vi "pl1000SetInterval.vi"(0 "pl1000 handle":i16, 5 "usForBlock":u32, 7 "idealNoOfSamples":u32, 9 "channels":i16[](array[numeric]), 11 "error in (no error)":errorcluster) -> (4 "pl1000 handle out":i16, 6 "usForBlock OP":u32, 8 "idealNoOfSamples OP":u32, 15 "error out":errorcluster)   [LabVIEW 2010]
doc: "This function sets the sampling rate of the unit. The fastest possible sampling interval is 1 microsecond, when the number of samples\nis 8192 divided by the number of channels active and the capture mode is BM_SINGLE. Under all other conditions, the fastest possible sampling interval is 10 microseconds per channel. The fastest possible data collection in the streaming settings is 100 kS/s (10 µs per sample), shared across all channels.\n\nus_for_block: target total time in which to collect\nideal_no_of_samples, in microseconds\n\nideal_no_of_samples: the total number of samples that you want\nto collect across all channels. This number is used only for timing\ncalculations\n\nchannels: an array of numbers identifying the channels from which\nyou wish to capture data"
uses:
  pl1000.dll
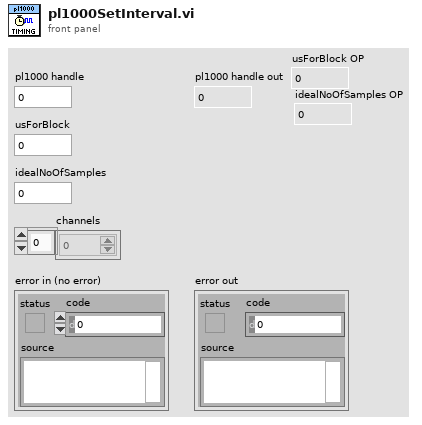
[diagram p1: front panel]
types:
  T1 = cluster{"status":bool, "code":u32, "source":string}
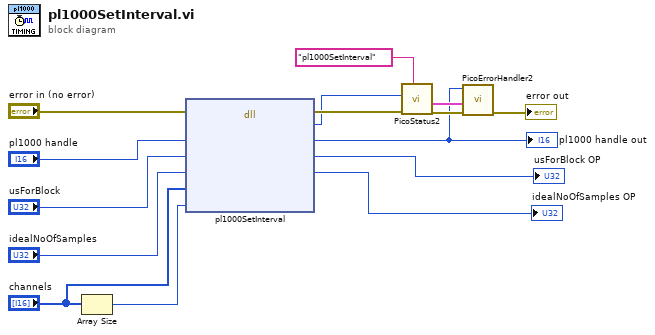
[diagram p0: block diagram]
diagram:
  n1 = Array Size(array="channels") -> (size(s)=w13:i32)
  n2 = dll-call lib="pl1000.dll" fn="pl1000SetInterval"(error in="error in (no error)", "handle"="pl1000 handle", "usForBlock"="usForBlock", "idealNoOfSamples"="idealNoOfSamples", "channels"="channels", "noOfChannels"=w13) -> (error out=w6:errorcluster, "status"=w5:u32, "handle"=w4:i16, "usForBlock"=→"usForBlock OP":u32, "idealNoOfSamples"=→"idealNoOfSamples OP":u32)  [unwired: 4 in, 1 out]
  "pl1000 handle out" <- w4
  n3 = call "PicoStatus2.vi"("PICO source"="pl1000SetInterval", "Error in"=w6, "PICO STATUS"=w5) -> ("error out"=w8:errorcluster, "PICO_STATUS out"=w7:T1)  [unwired: 5 in]
  n4 = call "PicoErrorHandler2.vi"("error in (no error)"=w8, "PICO_STATUS in"=w7, "handle In"=w4) -> ("error out"=→"error out":errorcluster)  [unwired: 8 in]
